vi "HFRR ADV v036.vi"() -> ()   [LabVIEW 2025] (continued)
          tunnel: [T19."Disabled" ("Disabled") T19."Enabled" ("Disabled")] -> w1363
          frame False {
          }
          frame True {
          }
        }
        n1482 = property on="About" class="Bool (strict)"("DisabledEnum"=w1363) -> ()  [unwired: 2 in, 2 out]
      }
      frame "Test Setup" {
        w1369 = T19."Enabled" ("Disabled")
        n1483 = local read "Service Password enable"() -> (w1368:bool)
        n1484 = property on="Dashboard" class="Bool (strict)"("DisabledEnum"=T19."Disabled" ("Disabled")) -> ()  [unwired: 2 in, 2 out]
        n1485 = property on="Imaging" class="Bool (strict)"("DisabledEnum"=w1369) -> ()  [unwired: 2 in, 2 out]
        n1486 = property on="Analysis" class="Bool (strict)"("DisabledEnum"=w1369) -> ()  [unwired: 2 in, 2 out]
        n1487 = property on="Home" class="Bool (strict)"("DisabledEnum"=w1369) -> ()  [unwired: 2 in, 2 out]
        n1488 = property on="Report" class="Bool (strict)"("DisabledEnum"=w1369) -> ()  [unwired: 2 in, 2 out]
        n1489 = property on="Test Setup" class="Bool (strict)"("DisabledEnum"=w1369) -> ()  [unwired: 2 in, 2 out]
        n1490 = case shown="True" w1368 {
          tunnel: [T19."Disabled" ("Disabled") T19."Enabled" ("Disabled")] -> w1367
          frame False {
          }
          frame True {
          }
        }
        n1491 = property on="About" class="Bool (strict)"("DisabledEnum"=w1367) -> ()  [unwired: 2 in, 2 out]
      }
      frame "Adv Scar" {
        w1376 = T19."Enabled" ("Disabled")
        n1492 = property on="Dashboard" class="Bool (strict)"("DisabledEnum"=T19."Disabled" ("Disabled")) -> ()  [unwired: 2 in, 2 out]
        n1493 = property on="Imaging" class="Bool (strict)"("DisabledEnum"=w1376) -> ()  [unwired: 2 in, 2 out]
        n1494 = property on="Analysis" class="Bool (strict)"("DisabledEnum"=w1376) -> ()  [unwired: 2 in, 2 out]
        n1495 = property on="Home" class="Bool (strict)"("DisabledEnum"=w1376) -> ()  [unwired: 2 in, 2 out]
        n1496 = property on="Report" class="Bool (strict)"("DisabledEnum"=w1376) -> ()  [unwired: 2 in, 2 out]
        n1497 = property on="Test Setup" class="Bool (strict)"("DisabledEnum"=w1376) -> ()  [unwired: 2 in, 2 out]
        n1498 = local read "Service Password enable"() -> (w1374:bool)
        n1499 = case shown="True" w1374 {
          tunnel: [T19."Disabled" ("Disabled") T19."Enabled" ("Disabled")] -> w1373
          frame False {
          }
          frame True {
          }
        }
        n1500 = property on="About" class="Bool (strict)"("DisabledEnum"=w1373) -> ()  [unwired: 2 in, 2 out]
      }
      frame "Calibration" {
        w1379 = T19."Enabled" ("Disabled")
        n1501 = property on="Dashboard" class="Bool (strict)"("DisabledEnum"=T19."Disabled" ("Disabled")) -> ()  [unwired: 2 in, 2 out]
        n1502 = property on="Imaging" class="Bool (strict)"("DisabledEnum"=w1379) -> ()  [unwired: 2 in, 2 out]
        n1503 = property on="Analysis" class="Bool (strict)"("DisabledEnum"=w1379) -> ()  [unwired: 2 in, 2 out]
        n1504 = property on="Home" class="Bool (strict)"("DisabledEnum"=w1379) -> ()  [unwired: 2 in, 2 out]
        n1505 = property on="Report" class="Bool (strict)"("DisabledEnum"=w1379) -> ()  [unwired: 2 in, 2 out]
        n1506 = property on="Test Setup" class="Bool (strict)"("DisabledEnum"=w1379) -> ()  [unwired: 2 in, 2 out]
        n1507 = local read "Service Password enable"() -> (w1381:bool)
        n1508 = property on="Calibration" class="Bool (strict)"("DisabledEnum"=w1379) -> ()  [unwired: 2 in, 2 out]
        n1509 = case shown="True" w1381 {
          tunnel: [T19."Disabled" ("Disabled") T19."Enabled" ("Disabled")] -> w1380
          frame False {
          }
          frame True {
          }
        }
        n1510 = property on="About" class="Bool (strict)"("DisabledEnum"=w1380) -> ()  [unwired: 2 in, 2 out]
      }
      frame "Adv Scar Report" {
        w1387 = T19."Enabled" ("Disabled")
        n1511 = property on="Dashboard" class="Bool (strict)"("DisabledEnum"=T19."Disabled" ("Disabled")) -> ()  [unwired: 2 in, 2 out]
        n1512 = property on="Imaging" class="Bool (strict)"("DisabledEnum"=w1387) -> ()  [unwired: 2 in, 2 out]
        n1513 = property on="Analysis" class="Bool (strict)"("DisabledEnum"=w1387) -> ()  [unwired: 2 in, 2 out]
        n1514 = property on="Home" class="Bool (strict)"("DisabledEnum"=w1387) -> ()  [unwired: 2 in, 2 out]
        n1515 = property on="Report" class="Bool (strict)"("DisabledEnum"=w1387) -> ()  [unwired: 2 in, 2 out]
        n1516 = property on="Test Setup" class="Bool (strict)"("DisabledEnum"=w1387) -> ()  [unwired: 2 in, 2 out]
        n1517 = local read "Service Password enable"() -> (w1386:bool)
        n1518 = case shown="True" w1386 {
          tunnel: [T19."Disabled" ("Disabled") T19."Enabled" ("Disabled")] -> w1385
          frame False {
          }
          frame True {
          }
        }
        n1519 = property on="About" class="Bool (strict)"("DisabledEnum"=w1385) -> ()  [unwired: 2 in, 2 out]
      }
      frame "Compare Files" {
        w1393 = T19."Enabled" ("Disabled")
        n1520 = local read "Service Password enable"() -> (w1392:bool)
        n1521 = property on="Dashboard" class="Bool (strict)"("DisabledEnum"=T19."Disabled" ("Disabled")) -> ()  [unwired: 2 in, 2 out]
        n1522 = property on="Imaging" class="Bool (strict)"("DisabledEnum"=w1393) -> ()  [unwired: 2 in, 2 out]
        n1523 = property on="Analysis" class="Bool (strict)"("DisabledEnum"=w1393) -> ()  [unwired: 2 in, 2 out]
        n1524 = property on="Home" class="Bool (strict)"("DisabledEnum"=w1393) -> ()  [unwired: 2 in, 2 out]
        n1525 = property on="Report" class="Bool (strict)"("DisabledEnum"=w1393) -> ()  [unwired: 2 in, 2 out]
        n1526 = property on="Test Setup" class="Bool (strict)"("DisabledEnum"=w1393) -> ()  [unwired: 2 in, 2 out]
        n1527 = case shown="True" w1392 {
          tunnel: [T19."Disabled" ("Disabled") T19."Enabled" ("Disabled")] -> w1391
          frame False {
          }
          frame True {
          }
        }
        n1528 = property on="About" class="Bool (strict)"("DisabledEnum"=w1391) -> ()  [unwired: 2 in, 2 out]
      }
      frame "Acquire" {
        n1529 = local read "Service Password enable"() -> (w1398:bool)
        n1530 = property on="Test Setup" class="Bool (strict)"("DisabledEnum"=T19."Disabled" ("Disabled")) -> ()  [unwired: 2 in, 2 out]
        n1531 = local read "Auto Start Test"() -> (w1400:bool)
        n1532 = local read "RUN"() -> (w1402:bool)
        n1533 = case shown="True" w1398 {
          tunnel: [T19."Disabled" ("Disabled") T19."Enabled" ("Disabled")] -> w1399
          frame False {
          }
          frame True {
          }
        }
        n1534 = Or(x=w1402, y=w1400) -> (x .or. y?=w1401:bool)
        n1535 = case shown="True" w1401 {
          tunnel: [T19."Enabled" ("Disabled") T19."Disabled" ("Disabled")] -> w1397
          frame False {
          }
          frame True {
          }
        }
        n1536 = property on="About" class="Bool (strict)"("DisabledEnum"=w1399) -> ()  [unwired: 2 in, 2 out]
        n1537 = property on="Imaging" class="Bool (strict)"("DisabledEnum"=w1397) -> ()  [unwired: 2 in, 2 out]
        n1538 = property on="Dashboard" class="Bool (strict)"("DisabledEnum"=w1397) -> ()  [unwired: 2 in, 2 out]
        n1539 = property on="Analysis" class="Bool (strict)"("DisabledEnum"=w1397) -> ()  [unwired: 2 in, 2 out]
        n1540 = property on="Home" class="Bool (strict)"("DisabledEnum"=w1397) -> ()  [unwired: 2 in, 2 out]
        n1541 = property on="Report" class="Bool (strict)"("DisabledEnum"=w1397) -> ()  [unwired: 2 in, 2 out]
        n1542 = property on="Calibration" class="Bool (strict)"("DisabledEnum"=w1397) -> ()  [unwired: 2 in, 2 out]
      }
      frame "About" {
        n1543 = local read "FILE"() -> (w1416:string)
        n1544 = local read "TEST FILE NAM,E SAVED"() -> (w1409:bool)
        n1545 = call <vilib>:"Trim Whitespace.vi"("string"=w1416) -> ("trimmed string"=w1415:string)  [unwired: 1 in]
        n1546 = local read "Auto Start Test"() -> (w1419:bool)
        n1547 = String Length(string=w1415) -> (length=w1414:i32)
        n1548 = Greater?(x=w1414, y=1) -> (0:w1411:bool)
        n1549 = And(x=w1411, y=w1409) -> (x .and. y?=w1410:bool)
        n1550 = local read "RUN"() -> (w1421:bool)
        n1551 = case shown="True" w1410 {
          tunnel: [T19."Disabled" ("Disabled") T19."Enabled" ("Disabled")] -> w1412
          frame False {
          }
          frame True {
          }
        }
        n1552 = Or(x=w1421, y=w1419) -> (x .or. y?=w1420:bool)
        n1553 = property on="About" class="Bool (strict)"("DisabledEnum"=T19."Enabled" ("Disabled")) -> ()  [unwired: 2 in, 2 out]
        n1554 = case shown="False" w1420 {
          tunnel: [T19."Enabled" ("Disabled") T19."Disabled" ("Disabled")] -> w1418
          frame False {
          }
          frame True {
          }
        }
        n1555 = property on="Dashboard" class="Bool (strict)"("DisabledEnum"=w1412) -> ()  [unwired: 2 in, 2 out]
        n1556 = property on="Test Setup" class="Bool (strict)"("DisabledEnum"=T19."Disabled" ("Disabled")) -> ()  [unwired: 2 in, 2 out]
        n1557 = property on="Imaging" class="Bool (strict)"("DisabledEnum"=w1418) -> ()  [unwired: 2 in, 2 out]
        n1558 = property on="Analysis" class="Bool (strict)"("DisabledEnum"=w1418) -> ()  [unwired: 2 in, 2 out]
        n1559 = property on="Home" class="Bool (strict)"("DisabledEnum"=w1418) -> ()  [unwired: 2 in, 2 out]
        n1560 = property on="Report" class="Bool (strict)"("DisabledEnum"=w1418) -> ()  [unwired: 2 in, 2 out]
      }
    }
    n1561 = local read "Quit"() -> (w1346:bool)
    "Single" <- "Single - Graph"
  }
  n1562 = disable-structure shown="Disabled" {
    disable-tunnel: [w1698 _] -> w42
    disable-tunnel: _ -> [w1697 _]
    frame Disabled {
      n1563 = while {
        tunnel: w1697 -> [_]
        tunnel: [w1699] -> w1698
        tunnel: [w1700] -> _
        i -> [w1700]
        stop <- w1699 stop-if-true
        w1716 = u16 10 items=["1.0"=10, "1.5"=15, "2.0"=20] ("stop bits (10: 1 bit)")
        n1564 = Wait (ms)(milliseconds to wait=u32 10) -> ()  [unwired: 1 out]
        n1565 = call-poly "VISA Configure Serial Port"("VISA resource name"=refnum<visa-resource-name> "ASRL1::INSTR" ("COM PORT"), "timeout (10sec)"=u32 10, "baud rate (9600)"=u32 57600, "data bits (8)"=u16 8, "stop bits (10: 1 bit)"=w1716) -> ("VISA resource name out"=w1702:refnum<visa-resource-name>, "error out"=w1711:errorcluster)  [unwired: 9 in]
        n1566 = VISA Read(VISA resource name=w1702, byte count=u32 2 ("byte count (0)")) -> (read buffer=w1710:string)  [unwired: 1 in, 3 out]
        n1567 = String Subset(string=w1710, offset (0)=0, length (rest)=2 ("length (rest)")) -> (substring=w1709:string)
        n1568 = Match Pattern(string=w1709, regular expression="<>") -> (offset past match=w1706:i32)  [unwired: 1 in, 3 out]
        n1569 = Greater Or Equal?(x=w1706, y=0) -> (x >= y?=w1701:bool)
        n1570 = case shown="True" w1701 {
          tunnel: w1702 -> [_ w1720]
          tunnel: w1711 -> [_ w1719]
          frame False {
          }
          frame True {
            n1571 = VISA Read(VISA resource name=w1720, byte count=u32 32 ("byte count (0)"), error in (no error)=w1719) -> (read buffer=w1718:string)  [unwired: 3 out]
            n1572 = String Subset(string=w1718, offset (0)=0, length (rest)=8 ("length (rest)")) -> (substring=w1722:string)
            n1573 = String Subset(string=w1718, offset (0)=8, length (rest)=8 ("length (rest)")) -> (substring=w1723:string)
            n1574 = Decimal String To Number(string=w1723) -> (number=w1730:i32)  [unwired: 2 in, 1 out]
            n1575 = Decimal String To Number(string=w1722) -> (number=w1726:i32)  [unwired: 2 in, 1 out]
            n1576 = Divide(x=w1730, y=10000) -> ()  [unwired: 1 out]
            n1577 = Divide(x=w1726, y=1000000) -> ()  [unwired: 1 out]
          }
        }
        n1578 = local read "Quit"() -> (w1699:bool)
      }
    }
    frame Enabled {
    }
  }
  n1579 = Tick Count (ms)() -> (millisecond timer value=w4:u32)
  n1580 = while {
    shift-right: [w1776] -> _
    shift-left: w6 -> [w1780]
    shift-right: [w1775] -> _
    shift-left: w5 -> [w1779]
    shift-right: [w1774] -> _
    shift-left: w6 -> [w1778]
    shift-right: [w1773] -> _
    shift-left: w5 -> [w1777]
    shift-right: [w1771] -> _
    shift-left: w4 -> [w1772]
    shift-right: [w1768] -> _
    shift-left: w3 -> [w1769]
    shift-right: [w1767] -> _
    shift-left: w3 -> [w1770]
    shift-right: [w1760] -> _
    shift-left: w3 -> [w1766]
    shift-right: [w1759] -> _
    shift-left: w3 -> [w1765]
    shift-right: [w1758] -> _
    shift-left: w3 -> [w1764]
    shift-right: [w1757] -> _
    shift-left: w3 -> [w1763]
    shift-right: [w1756] -> _
    shift-left: w3 -> [w1762]
    shift-right: [w1755] -> _
    shift-left: w3 -> [w1761]
    shift-right: [w1754] -> _
    shift-left: w3 -> [w1748]
    shift-right: [w1753] -> _
    shift-left: w3 -> [w1747]
    shift-right: [w1752] -> _
    shift-left: w3 -> [w1746]
    shift-right: [w1751] -> _
    shift-left: w3 -> [w1745]
    shift-right: [w1750] -> _
    shift-left: w3 -> [w1744]
    shift-right: [w1749] -> _
    shift-left: w3 -> [w1743]
    shift-right: [w1734] -> _
    shift-left: w3 -> [w1737]
    shift-right: [w1733] -> _
    shift-left: w3 -> [w1736]
    shift-right: [w1732] -> _
    shift-left: w3 -> [w1735]
    stop <- w1782 stop-if-true
    n1581 = local read "Read UNO"() -> (w1741:string)
    n1582 = local read "Error  2"() -> (w1781:errorcluster)
    n1583 = String Length(string=w1741) -> (length=w1740:i32)
    n1584 = call <vilib>:"Trim Whitespace.vi"("string"=w1741) -> ("trimmed string"=w1742:string)  [unwired: 1 in]
    n1585 = Greater Or Equal?(x=w1740, y=23) -> (x >= y?=w1738:bool)
    n1586 = case shown="No Error" w1781 {
      tunnel: w1780 -> [w1828 w1924]
      tunnel: w1779 -> [w1827 w1923]
      tunnel: w1778 -> [w1826 w1922]
      tunnel: w1777 -> [w1825 w1921]
      tunnel: [w1824 w1924] -> w1776
      tunnel: [w1823 w1923] -> w1775
      tunnel: [w1822 w1922] -> w1774
      tunnel: [w1821 w1921] -> w1773
      tunnel: w1772 -> [w1820 w1920]
      tunnel: [w1819 w1920] -> w1771
      tunnel: w1769 -> [w1818 w1919]
      tunnel: w1770 -> [w1817 w1918]
      tunnel: [w1816 w1919] -> w1768
      tunnel: [w1815 w1918] -> w1767
      tunnel: w1766 -> [w1814 w1917]
      tunnel: w1765 -> [w1813 w1916]
      tunnel: w1764 -> [w1812 w1915]
      tunnel: w1763 -> [w1811 w1914]
      tunnel: w1762 -> [w1810 w1913]
      tunnel: w1761 -> [w1809 w1912]
      tunnel: [w1808 w1917] -> w1760
      tunnel: [w1807 w1916] -> w1759
      tunnel: [w1806 w1915] -> w1758
      tunnel: [w1805 w1914] -> w1757
      tunnel: [w1804 w1913] -> w1756
      tunnel: [w1803 w1912] -> w1755
      tunnel: w1748 -> [w1802 w1911]
      tunnel: [w1801 w1911] -> w1754
      tunnel: [w1800 w1907] -> w1753
      tunnel: [w1799 w1906] -> w1752
      tunnel: [w1798 w1910] -> w1751
      tunnel: [w1797 w1909] -> w1750
      tunnel: [w1796 w1908] -> w1749
      tunnel: w1747 -> [w1795 w1910]
      tunnel: w1746 -> [w1794 w1909]
      tunnel: w1745 -> [w1793 w1908]
      tunnel: w1744 -> [w1792 w1907]
      tunnel: w1743 -> [w1791 w1906]
      tunnel: w1742 -> [w1790 _]
      tunnel: w1738 -> [w1789 _]
      tunnel: w1737 -> [w1788 w1905]
      tunnel: w1736 -> [w1787 w1904]
      tunnel: w1735 -> [w1786 w1903]
      tunnel: [w1785 w1905] -> w1734
      tunnel: [w1784 w1904] -> w1733
      tunnel: [w1783 w1903] -> w1732
      frame No Error {
        n1587 = case shown="True" w1789 {
          tunnel: w1828 -> [w1844 w1896]
          tunnel: w1827 -> [w1843 w1895]
          tunnel: w1826 -> [w1842 w1894]
          tunnel: w1825 -> [w1841 w1893]
          tunnel: [w1844 w1892] -> w1824
          tunnel: [w1843 w1891] -> w1823
          tunnel: [w1842 w1890] -> w1822
          tunnel: [w1841 w1889] -> w1821
          tunnel: w1820 -> [w1840 w1887]
          tunnel: [w1840 w1886] -> w1819
          tunnel: w1818 -> [w1839 w1885]
          tunnel: w1817 -> [w1838 w1884]
          tunnel: [w1839 w1883] -> w1816
          tunnel: [w1838 w1882] -> w1815
          tunnel: w1814 -> [w1837 w1881]
          tunnel: w1813 -> [w1836 w1880]
          tunnel: w1812 -> [w1835 w1879]
          tunnel: w1811 -> [w1834 w1878]
          tunnel: w1810 -> [w1833 w1877]
          tunnel: w1809 -> [w1832 w1876]
          tunnel: [w1837 w1875] -> w1808
          tunnel: [w1836 w1874] -> w1807
          tunnel: [w1835 w1873] -> w1806
          tunnel: [w1834 w1872] -> w1805
          tunnel: [w1833 w1871] -> w1804
          tunnel: [w1832 w1870] -> w1803
          tunnel: w1802 -> [w1850 w1869]
          tunnel: [w1850 w1868] -> w1801
          tunnel: [w1847 w1867] -> w1800
          tunnel: [w1846 w1866] -> w1799
          tunnel: [w1849 w1865] -> w1798
          tunnel: [w1845 w1864] -> w1797
          tunnel: [w1848 w1863] -> w1796
          tunnel: w1795 -> [w1849 w1862]
          tunnel: w1794 -> [w1848 w1861]
          tunnel: w1793 -> [w1847 w1860]
          tunnel: w1792 -> [w1846 w1859]
          tunnel: w1791 -> [w1845 w1858]
          tunnel: w1790 -> [_ w1857]
          tunnel: w1788 -> [w1831 w1856]
          tunnel: w1787 -> [w1830 w1855]
          tunnel: w1786 -> [w1829 w1854]
          tunnel: [w1831 w1853] -> w1785
          tunnel: [w1830 w1852] -> w1784
          tunnel: [w1829 w1851] -> w1783
          frame False {
          }
          frame True {
            n1588 = Tick Count (ms)() -> (millisecond timer value=w1888:u32)
            n1589 = String To Byte Array(string=w1857) -> (unsigned byte array=w1901:u8[])
            n1590 = Array Size(array=w1901) -> (size(s)=w1900:i32)
            n1591 = formula code="// --- INTERNAL VARIABLE DECLARATIONS ---\nint i = 0;\nint k = 0;\nint start_idx = -1;\nint end_idx = -1;\nint phase = 0;\nint sign0 = 1;\nint sign1 = 1;\nint ch0_val = 0;   \nint ch1_val = 0;   \nfloat ch0_raw = 0.0;\nfloat ch1_raw = 0.0;\nfloat temp0 = 0.0;\nfloat temp1 = 0.0;\nfloat ch0_clean = 0.0;\nfloat ch1_clean = 0.0;\n\nint valid_samples = 0; // FIX: Track if we actually parsed new data this window\nfloat max_allowed_bits = 8388607.0; // FIX: Change this to match your ADC max value\n\n// Temporal intermediate variables for calculation smoothing\nfloat raw_p2p_v = 0.0;\nfloat raw_friction = 0.0;\nfloat raw_cof = 0.0;\n\n// Temporal intermediate variables for Piezo voltage translations\nfloat piezo_min_v = 0.0;\nfloat piezo_max_v = 0.0;\n\n// Initialize output variables to current shift register states right away\nout_LVDT_Min_V = in_LVDT_Min_V;\nout_LVDT_Max_V = in_LVDT_Max_V;\nout_LVDT_P2P_V = in_LVDT_P2P_V;\nout_Piezo_P2P = in_Piezo_P2P;\nout_Friction_N = in_Friction_N;\nout_COF = in_COF;\nwindow_ready = 0;\n\n// --- STEP 1: PARSE EVERY STRING IN THE BYTE ARRAY ---\nif (array_size > 2) {\n    for (i = 0; i < array_size - 1; i++) {\n        if (raw_bytes[i] == 42) { // '*' character detected\n            start_idx = i;\n        }\n        \n        // Match standard delimiter sequence \";&\" or end window character\n        if (raw_bytes[i] == 59 && raw_bytes[i+1] == 38 && start_idx != -1) { \n            end_idx = i;\n            ch0_val = 0;\n            ch1_val = 0;\n            sign0 = 1;\n            sign1 = 1;\n            phase = 0; \n\n            for (k = start_idx + 1; k < end_idx; k++) {\n                if (raw_bytes[k] == 45) { // '-' sign\n                    if (phase == 0) sign0 = -1;\n                    else sign1 = -1;\n                }\n                else if (raw_bytes[k] == 43) { // '+' sign\n                    if (phase == 0) sign0 = 1;\n                    else sign1 = 1;\n                }\n                else if (raw_bytes[k] == 59) { // ';' delimiter\n                    phase = 1; \n                }\n                else if (raw_bytes[k] >= 48 && raw_bytes[k] <= 57) { // Numeric ASCII digits\n                    if (phase == 0) {\n                        ch0_val = (ch0_val * 10) + (raw_bytes[k] - 48);\n                    } else {\n                        ch1_val = (ch1_val * 10) + (raw_bytes[k] - 48);\n                    }\n                }\n            }\n\n            // Implicit type conversion\n            ch0_raw = ch0_val * sign0 * 1.0;\n            ch1_raw = ch1_val * sign1 * 1.0;\n\n            // FIX: Sanity check / Hard-clamping to catch sudden massive ASCII noise spikes\n            if (ch0_raw > max_allowed_bits)  ch0_raw = max_allowed_bits;\n            if (ch0_raw < -max_allowed_bits) ch0_raw = -max_allowed_bits;\n            if (ch1_raw > max_allowed_bits)  ch1_raw = max_allowed_bits;\n            if (ch1_raw < -max_allowed_bits) ch1_raw = -max_allowed_bits;\n\n            // --- STEP 2: 3-SAMPLE MEDIAN FILTER ---\n            m0_2 = m0_1; m0_1 = m0_0; m0_0 = ch0_raw;\n            float s0_0 = m0_0; float s0_1 = m0_1; float s0_2 = m0_2;\n            if (s0_0 > s0_1) { temp0 = s0_0; s0_0 = s0_1; s0_1 = temp0; }\n            if (s0_1 > s0_2) { temp0 = s0_1; s0_1 = s0_2; s0_2 = temp0; }\n            if (s0_0 > s0_1) { temp0 = s0_0; s0_0 = s0_1; s0_1 = temp0; }\n            ch0_clean = s0_1;\n\n            m1_2 = m1_1; m1_1 = m1_0; m1_0 = ch1_raw;\n            float s1_0 = m1_0; float s1_1 = m1_1; float s1_2 = m1_2;\n            if (s1_0 > s1_1) { temp1 = s1_0; s1_0 = s1_1; s1_1 = temp1; }\n            if (s1_1 > s1_2) { temp1 = s1_1; s1_1 = s1_2; s1_2 = temp1; }\n            if (s1_0 > s1_1) { temp1 = s1_0; s1_0 = s1_1; s1_1 = temp1; }\n            ch1_clean = s1_1;\n\n            // --- STEP 3: EXPONENTIAL FILTER (STREAM LEVEL) ---\n            if (ch0_filt == 0.0) ch0_filt = ch0_clean;\n            if (ch1_filt == 0.0) ch1_filt = ch1_clean;\n\n            ch0_filt = ch0_filt + (ch0_clean - ch0_filt) * 0.125;\n            ch1_filt = ch1_filt + (ch1_clean - ch1_filt) * 0.125;\n\n            // --- STEP 4: MIN/MAX WINDOW CONTINUOUS ACCUMULATION ---\n            if (ch0_filt > max_ch0) max_ch0 = ch0_filt;\n            if (ch0_filt < min_ch0) min_ch0 = ch0_filt;\n            if (ch1_filt > max_ch1) max_ch1 = ch1_filt;\n            if (ch1_filt < min_ch1) min_ch1 = ch1_filt;\n\n            valid_samples++; // FIX: Successfully parsed and accumulated a clean point\n            start_idx = -1; \n        }\n    }\n}\n\n// --- STEP 5: WINDOW EVALUATION ENGINE ---\n// FIX: Condition updated to verify that valid samples exist for both channels\nif (((current_time_ms - start_time_ms) >= 50) && (valid_samples > 0) && (min_ch0 < 9000000.0) && (min_ch1 < 9000000.0)) {\n    window_ready = 1;\n\n    // Linear Bit-to-Voltage Transformations (LVDT - Channel 0)\n    out_LVDT_Min_V = (min_ch0 * VREF) / 8388607.0;\n    out_LVDT_Max_V = (max_ch0 * VREF) / 8388607.0;\n    raw_p2p_v = out_LVDT_Max_V - out_LVDT_Min_V;\n\n    // Linear Bit-to-Voltage Transformations (Piezo - Channel 1)\n    piezo_min_v = (min_ch1 * VREF) / 8388607.0;\n    piezo_max_v = (max_ch1 * VREF) / 8388607.0;\n    \n    // Assign Peak-to-Peak Voltage directly to output indicator (Matches Python logic)\n    out_Piezo_P2P = piezo_max_v - piezo_min_v;\n    \n    // Force scaling calculations using Voltage delta * Newtons/Volt Factor\n    raw_friction = out_Piezo_P2P * PIEZO_CAL_FACTOR + 0.44528;\n    raw_cof = raw_friction / NORMAL_FORCE;\n\n    // --- STEP 6: OUTPUT METRIC SMOOTHING (Low-Pass Filter Alpha = 0.05) ---\n    // Seed initial historical metrics if first loop iteration\n    if (hist_LVDT_P2P == 0.0) hist_LVDT_P2P = raw_p2p_v;\n    if (hist_Friction == 0.0) hist_Friction = raw_friction;\n    if (hist_COF == 0.0)      hist_COF = raw_cof;\n\n    // Apply exponential output dampening\n    hist_LVDT_P2P = hist_LVDT_P2P + (raw_p2p_v - hist_LVDT_P2P) * 0.05;\n    hist_Friction = hist_Friction + (raw_friction - hist_Friction) * 0.05; // Note: Can drop to 0.02 for more aggressive damping\n    hist_COF      = hist_COF + (raw_cof - hist_COF) * 0.05;\n\n    // Direct smoothed parameters out to UI Indicators\n    out_LVDT_P2P_V = hist_LVDT_P2P;\n    out_Friction_N = hist_Friction;\n    out_COF        = hist_COF;\n\n    // Reset tracking targets to extreme boundaries safely\n    min_ch0 = 9999999.0;\n    max_ch0 = -9999999.0;\n    min_ch1 = 9999999.0;\n    max_ch1 = -9999999.0;\n\n    valid_samples = 0; // FIX: Reset counter for next time frame\n    start_time_ms = current_time_ms;\n}"("raw_bytes"=w1901, "array_size"=w1900, "VREF"="VREF", "PIEZO_CAL_FACTOR"="PIEZO_CAL_FACTOR", "NORMAL_FORCE"="NORMAL_FORCE", "min_ch0"=w1896, "max_ch0"=w1895, "min_ch1"=w1894, "max_ch1"=w1893, "current_time_ms"=w1888, "start_time_ms"=w1887, "ch0_filt"=w1885, "ch1_filt"=w1884, "m0_0"=w1881, "m0_1"=w1880, "m0_2"=w1879, "m1_0"=w1878, "m1_1"=w1877, "m1_2"=w1876, "in_LVDT_Min_V"=w1869, "in_LVDT_Max_V"=w1862, "in_LVDT_P2P_V"=w1861, "in_Piezo_P2P"=w1860, "in_Friction_N"=w1859, "in_COF"=w1858, "hist_LVDT_P2P"=w1856, "hist_Friction"=w1855, "hist_COF"=w1854) -> ("window_ready"=→"Valid_data":dbl, "out_LVDT_Min_V"=w1868:dbl, "out_LVDT_Max_V"=w1867:dbl, "out_LVDT_P2P_V"=w1866:dbl, "out_Piezo_P2P"=w1865:dbl, "out_Friction_N"=w1864:dbl, "out_COF"=w1863:dbl, "min_ch0"=w1892:dbl, "max_ch0"=w1891:dbl, "min_ch1"=w1890:dbl, "max_ch1"=w1889:dbl, "start_time_ms"=w1886:u32, "ch0_filt"=w1883:dbl, "ch1_filt"=w1882:dbl, "m0_0"=w1875:dbl, "m0_1"=w1874:dbl, "m0_2"=w1873:dbl, "m1_0"=w1872:dbl, "m1_1"=w1871:dbl, "m1_2"=w1870:dbl, "hist_LVDT_P2P"=w1853:dbl, "hist_Friction"=w1852:dbl, "hist_COF"=w1851:dbl)
            "LVDT MIN" <- w1868
            "LVDT MAX" <- w1867
            "LVDT Peak" <- w1866
            "pizo raw" <- w1865
            "cof" <- w1863
            "Frictioin Force Raw" <- w1864
          }
        }
      }
      frame Error {
      }
    }
    n1592 = local read "Quit"() -> (w1782:bool)
  }
  n1593 = disable-structure shown="Disabled" {
    disable-tunnel: errorcluster {"status"=TRUE, "code"=0, "source"="Init"} ("error IO") -> [w1927 _]
    disable-tunnel: [w1925 _] -> w45
    frame Disabled {
      n1594 = while {
        shift-right: [w1943] -> w1929
        shift-left: _ -> [w1934]
        shift-right: [w1942] -> w1928
        shift-left: w1927 -> [w1936]
        tunnel: [w1931] -> w1925
        tunnel: [w1941] -> _
        i -> [w1941]
        stop <- w1931 stop-if-true
        n1595 = local read "Port 1a"() -> (w1937:bool)
        n1596 = local read "Port 3"() -> (w1938:bool)
        n1597 = local read "Com Port 1"() -> (w1935:refnum<visa-resource-name>)
        n1598 = Or(x=w1938, y=w1937) -> (x .or. y?=w1940:bool)
        n1599 = Unbundle(w1936) -> ("status"=→"Port 3":bool)  [unwired: 2 out]
        n1600 = Not Equal?(x=w1935, y=w1934) -> (x != y?=w1932:bool)
        n1601 = case shown="True" w1940 {
          frame False {
            w1946 = TRUE ("Visible")
            n1602 = property on="Port 1a" class="Bool (strict)"("Visible"=w1946) -> ()  [unwired: 2 in, 2 out]
            n1603 = property on="Port 3" class="Bool (strict)"("Visible"=w1946) -> ()  [unwired: 2 in, 2 out]
          }
          frame True {
            w1947 = TRUE ("Visible")
            n1604 = property on="Port 1a" class="Bool (strict)"("Visible"=w1947) -> ()  [unwired: 2 in, 2 out]
            n1605 = property on="Port 3" class="Bool (strict)"("Visible"=w1947) -> ()  [unwired: 2 in, 2 out]
          }
        }
        n1606 = Wait (ms)(milliseconds to wait=u32 40) -> ()  [unwired: 1 out]
        n1607 = case shown="True" w1932 {
          tunnel: [w1944 errorcluster {"status"=TRUE, "code"=0, "source"="Init"} ("error out")] -> w1933
          tunnel: w1936 -> [w1944 _]
          frame False {
          }
          frame True {
          }
        }
        n1608 = case shown="Error" w1933 {
          selector: w1933 -> [w1954 w1972]
          tunnel: [w1957 w1976] -> w1943
          tunnel: [w1956 w1970] -> w1942
          tunnel: w1934 -> [w1955 w1974]
          frame No Error {
            n1609 = property class="Instr"(reference=w1955, error in=w1954) -> (reference out=w1952:refnum<visa-resource-name>, error out=w1953:errorcluster, "Serial Settings:Number of Bytes at Serial Port"=w1949:u32)
            n1610 = Greater?(x=w1949, y=u32 5) -> (0:w1948:bool)
            n1611 = Not(x=w1948) -> (.not. x?=→"Port 1a":bool)
            n1612 = while {
              tunnel: [w1965] -> w1956
              tunnel: [w1964] -> w1957
              tunnel: w1953 -> [w1963]
              tunnel: w1952 -> [w1962]
              stop <- TRUE stop-if-true
              n1613 = property class="Instr" props=["Serial Settings:Number of Bytes at Serial Port"](reference=w1962, error in=w1963) -> (reference out=w1967:refnum<visa-resource-name>, error out=w1966:errorcluster)  [unwired: 1 out]
              n1614 = VISA Read(VISA resource name=w1967, byte count=u32 50, error in (no error)=w1966) -> (VISA resource name out=w1964:refnum<visa-resource-name>, read buffer=w1959:string, error out=w1965:errorcluster)  [unwired: 1 out]
              n1615 = Wait (ms)(milliseconds to wait=u32 5) -> ()  [unwired: 1 out]
            }
          }
          frame Error {
            w1982 = u16 0 items=["None", "XON/XOFF", "RTS/CTS", "XON/XOFF & RTS/CTS", "DTR/DSR", "XON/XOFF & DTR/DSR"] ("flow control (0:none)  2")
            w1980 = u16 10 items=["1.0"=10, "1.5"=15, "2.0"=20] ("stop bits 2")
            w1978 = u16 0 items=["None", "Odd", "Even", "Mark", "Space"] ("parity 2")
            w1979 = u32 10000  # timeout (10sec)
            n1616 = VISA Close(VISA resource name=w1974, error in (no error)=w1972) -> (error out=w1975:errorcluster)
            n1617 = local write "Port 1a"(FALSE ("Port 1a")) -> ()
            n1618 = local read "Com Port 1"() -> (w1969:refnum<visa-resource-name>)
            n1619 = call <vilib>:"Clear Errors.vi"("error in (no error)"=w1975) -> ("error out"=w1973:errorcluster)  [unwired: 5 in, 1 out]
            n1620 = call-poly "VISA Configure Serial Port"("VISA resource name"=w1969, "timeout (10sec)"=w1979, "baud rate (9600)"=u32 250000 ("baud rate  2"), "data bits (8)"=u16 8 ("data bits  2"), "parity (0:none)"=w1978, "error in (no error)"=w1973, "stop bits (10: 1 bit)"=w1980, "flow control (0:none)"=w1982) -> ("VISA resource name out"=w1983:refnum<visa-resource-name>, "error out"=w1984:errorcluster)  [unwired: 6 in]
            n1621 = flat-sequence {
              tunnel: w1983 -> [w1986]
              tunnel: w1984 -> [w1985]
              tunnel: [w1986] -> w1976
              tunnel: [w1985] -> w1970
              frame #0 {
                n1622 = Wait (ms)(milliseconds to wait=u32 50) -> ()  [unwired: 1 out]
              }
            }
            "Residual Uno" <- ""
          }
        }
        n1623 = local read "Quit"() -> (w1931:bool)
        "Error Uno" <- w1936
      }
      n1624 = VISA Close(VISA resource name=w1929, error in (no error)=w1928) -> (error out=w1926:errorcluster)
      n1625 = call <vilib>:"Clear Errors.vi"("error in (no error)"=w1926) -> ()  [unwired: 5 in, 2 out]
    }
    frame Enabled {
    }
  }
  n1626 = while {
    stop <- w1997 stop-if-true
    # "V0OLTAGE TO STROKE (peice vise calibration)"
    n1627 = local read "LVDT MIN"() -> (w1989:dbl)
    n1628 = local read "LVDT Peak"() -> (w1988:dbl)
    n1629 = Wait (ms)(milliseconds to wait=u32 10) -> ()  [unwired: 1 out]
    n1630 = formula code="// Dynamic Parameterized Linear Interpolation Node\n// Inputs: vpp_val, voltages (Array), distances (Array)\n// Outputs: stroke\n\nint i = 0;\nint segments = 11; // 12 points make 11 interpolation segments\n\n// 1. Lower Boundary Clamp\nif (vpp_val <= voltages[0]) {\n    stroke = distances[0];\n}\n// 2. Upper Boundary Clamp\nelse if (vpp_val >= voltages[segments]) {\n    stroke = distances[segments];\n}\n// 3. Dynamic Segment Search Loop\nelse {\n    stroke = distances[0]; // Fallback baseline\n    for (i = 0; i < segments; i++) {\n        if (vpp_val >= voltages[i] && vpp_val <= voltages[i+1]) {\n            // Standard linear interpolation formula using array lookups\n            stroke = distances[i] + (vpp_val - voltages[i]) * (distances[i+1] - distances[i]) / (voltages[i+1] - voltages[i]);\n            break; // Segment found, safely exit the loop\n        }\n    }\n}"("vpp_val"=w1988, "voltages"="calibration values", "distances"="STROKE") -> ("stroke"=→"LVDT STROKE":dbl)
    n1631 = local read "Calibration Tare Value"() -> (w1993:dbl)
    n1632 = local read "Calibration Tare"() -> (w1991:bool)
    n1633 = Subtract(x=w1989, y=w1993) -> (x-y=→"LVDT STROKE  Calibration":dbl)
    n1634 = case shown="True" w1991 {
      selector: w1991 -> [_ w1999]
      tunnel: w1989 -> [_ w2000]
      frame False {
      }
      frame True {
        n1635 = Not(x=w1999) -> (.not. x?=w1998:bool)
        n1636 = local write "Calibration Tare"(w1998) -> ()
        "Calibration Tare Value" <- w2000
      }
    }
    n1637 = local read "Quit"() -> (w1997:bool)
  }
  n1638 = while {
    stop <- w2023 stop-if-true
    n1639 = local read "Due read"() -> (w2021:string)
    n1640 = call <vilib>:"High Resolution Polling Wait.vi"("seconds to wait"=0.02) -> ()  [unwired: 10 in, 1 out]
    n1641 = local read "Frictioin Force Raw"() -> (w2003:dbl)
    n1642 = Spreadsheet String To Array(delimiter (Tab)=";", format string="", spreadsheet string=w2021, array type (2D Dbl)=string[] []) -> (array=w2018:string[])
    n1643 = Fract/Exp String To Number(string=w2018) -> (number=w2017:dbl[])  [unwired: 3 in, 1 out]
    n1644 = call <vilib>:"Median Filter PtByPt.vi"("rank"=2, "x"=w2003) -> ("Filtered x"=→"Friction":dbl)  [unwired: 2 in, 1 out]
    n1645 = Index Array(array=w2017) -> (element #1=→"Sample Temperature":dbl, element #2=→"Target Sample Temperature":dbl, element #3=→"Current Duty Cycle":dbl, element #4=→"Ambient Temperature":dbl, element #5=→"Dac Status":dbl, element #6=→"Vpp":dbl, element #7=→"Active Error Code":dbl, element #8=→"Kp":dbl, element #9=→"Ki":dbl, element #10=→"Kd":dbl, element #11=→"SampleRaw":dbl, element #12=→"AmbRaw":dbl)  [unwired: 12 in]
    n1646 = local read "Quit"() -> (w2023:bool)
  }
  n1647 = while {
    shift-right: [w2037] -> w41
    shift-left: _ -> [w2029]
    shift-right: [w2024] -> w40
    shift-left: errorcluster {"status"=FALSE, "code"=0, "source"="Init"} ("error out") -> [w2031]
    tunnel: [w2026] -> w44
    tunnel: [w2036] -> _
    i -> [w2036]
    stop <- w2026 stop-if-true
    n1648 = local read "Com Port 2"() -> (w2030:refnum<visa-resource-name>)
    n1649 = local read "Port 2a"() -> (w2032:bool)
    n1650 = Unbundle(w2031) -> ("status"=→"Port 4":bool)  [unwired: 2 out]
    n1651 = call <vilib>:"High Resolution Polling Wait.vi"("seconds to wait"=0.02) -> ()  [unwired: 10 in, 1 out]
    n1652 = local read "Port 4"() -> (w2033:bool)
    n1653 = Not Equal?(x=w2030, y=w2029) -> (x != y?=w2028:bool)
    n1654 = Or(x=w2033, y=w2032) -> (x .or. y?=w2035:bool)
    n1655 = case shown="False" w2035 {
      frame False {
        w2040 = TRUE ("Visible")
        n1656 = property on="Port 2a" class="Bool (strict)"("Visible"=w2040) -> ()  [unwired: 2 in, 2 out]
        n1657 = property on="Port 4" class="Bool (strict)"("Visible"=w2040) -> ()  [unwired: 2 in, 2 out]
      }
      frame True {
        w2041 = TRUE ("Visible")
        n1658 = property on="Port 2a" class="Bool (strict)"("Visible"=w2041) -> ()  [unwired: 2 in, 2 out]
        n1659 = property on="Port 4" class="Bool (strict)"("Visible"=w2041) -> ()  [unwired: 2 in, 2 out]
      }
    }
    n1660 = case shown="True" w2028 {
      tunnel: [w2038 errorcluster {"status"=TRUE, "code"=0, "source"="Init"} ("error out")] -> w2027
      tunnel: w2031 -> [w2038 _]
      frame False {
      }
      frame True {
      }
    }
    n1661 = case shown="No Error" w2027 {
      selector: w2027 -> [w2054 w2085]
      tunnel: [w2047 w2090] -> w2037
      tunnel: [w2055 w2083] -> w2024
      tunnel: w2029 -> [w2056 w2088]
      frame No Error {
        n1662 = property class="Instr" props=["Serial Settings:Number of Bytes at Serial Port"](reference=w2056, error in=w2054) -> (reference out=w2048:refnum<visa-resource-name>, error out=w2053:errorcluster)  [unwired: 1 out]
        n1663 = while {
          tunnel: [w2064] -> w2049
          tunnel: [w2063] -> w2050
          tunnel: w2053 -> [w2062]
          tunnel: w2048 -> [w2061]
          tunnel: [w2060] -> _
          i -> [w2060]
          stop <- TRUE stop-if-true
          n1664 = property class="Instr" props=["Serial Settings:Number of Bytes at Serial Port"](reference=w2061, error in=w2062) -> (reference out=w2066:refnum<visa-resource-name>, error out=w2065:errorcluster)  [unwired: 1 out]
          n1665 = VISA Read(VISA resource name=w2066, byte count=u32 1000, error in (no error)=w2065) -> (VISA resource name out=w2063:refnum<visa-resource-name>, read buffer=→"Due read":string, error out=w2064:errorcluster)  [unwired: 1 out]
        }
        n1666 = local read "Due Write"() -> (w2046:string)
        n1667 = call <vilib>:"Trim Whitespace.vi"("string"=w2046) -> ("trimmed string"=w2045:string)  [unwired: 1 in]
        n1668 = Not Equal?(x=w2045, y="") -> (x != y?=w2051:bool)
        n1669 = VISA Flush I/O Buffer(VISA resource name=w2050) -> (VISA resource name out=w2043:refnum<visa-resource-name>, error out=→"error out 10":errorcluster)  [unwired: 2 in]
        n1670 = case shown="True" w2051 {
          tunnel: w2043 -> [w2068 w2073]
          tunnel: [w2068 w2077] -> w2047
          tunnel: w2049 -> [w2067 w2072]
          tunnel: [w2067 w2075] -> w2055
          tunnel: w2045 -> [_ w2071]
          tunnel: [_ w2074] -> _
          frame False {
            # "DATA  WRITE LOOP"
          }
          frame True {
            n1671 = Concatenate Strings(w2071, "\r\n") -> (w2070:string)
            n1672 = VISA Write(VISA resource name=w2073, write buffer=w2070, error in (no error)=w2072) -> (VISA resource name out=w2077:refnum<visa-resource-name>, return count=w2074:u32, error out=w2076:errorcluster)
            n1673 = flat-sequence {
              tunnel: w2076 -> [w2079]
              tunnel: [w2079] -> w2075
              frame #0 {
                n1674 = local write "Due Write"("" ("Command")) -> ()
                n1675 = Wait (ms)(milliseconds to wait=u32 5) -> ()  [unwired: 1 out]
              }
            }
          }
        }
        "Port 2a" <- TRUE ("Port 2a")
      }
      frame Error {
        w2096 = u16 0 items=["None", "XON/XOFF", "RTS/CTS", "XON/XOFF & RTS/CTS", "DTR/DSR", "XON/XOFF & DTR/DSR"] ("flow control (0:none)  2")
        w2094 = u16 10 items=["1.0"=10, "1.5"=15, "2.0"=20] ("stop bits 2")
        w2092 = u16 0 items=["None", "Odd", "Even", "Mark", "Space"] ("parity 2")
        w2093 = u32 10000  # timeout (10sec)
        n1676 = VISA Clear(VISA resource name=w2088, error in (no error)=w2085) -> (VISA resource name out=w2087:refnum<visa-resource-name>, error out=w2086:errorcluster)
        n1677 = VISA Close(VISA resource name=w2087, error in (no error)=w2086) -> (error out=w2089:errorcluster)
        n1678 = call <vilib>:"Clear Errors.vi"("error in (no error)"=w2089) -> ()  [unwired: 5 in, 2 out]
        n1679 = local write "Port 2a"(FALSE ("Port 2a")) -> ()
        n1680 = local read "Com Port 2"() -> (w2082:refnum<visa-resource-name>)
        "visa due" <- w2082
        n1681 = call-poly "VISA Configure Serial Port"("VISA resource name"=w2082, "timeout (10sec)"=w2093, "baud rate (9600)"=u32 250000 ("baud rate  2"), "data bits (8)"=u16 8 ("data bits  2"), "parity (0:none)"=w2092, "stop bits (10: 1 bit)"=w2094, "flow control (0:none)"=w2096) -> ("VISA resource name out"=w2097:refnum<visa-resource-name>, "error out"=w2098:errorcluster)  [unwired: 7 in]
        n1682 = flat-sequence {
          tunnel: w2097 -> [w2100]
          tunnel: w2098 -> [w2099]
          tunnel: [w2100] -> w2090
          tunnel: [w2099] -> w2083
          frame #0 {
            n1683 = Wait (ms)(milliseconds to wait=u32 50) -> ()  [unwired: 1 out]
          }
        }
        "Residual Due" <- ""
      }
    }
    "error out 9" <- w2024
    n1684 = local read "Quit"() -> (w2026:bool)
    "Error Due" <- w2031
  }
  n1685 = local write "FRICVALZ"(0.0 ("FRICVALZ")) -> ()
  n1686 = property on="RUN" class="Bool (strict)"("Visible"=TRUE) -> ()  [unwired: 2 in, 2 out]
  n1687 = while {
    tunnel: [w2115] -> _
    tunnel: [w2102] -> w54
    i -> [w2115]
    stop <- w2102 stop-if-true
    n1688 = local read "conststatus"() -> (w2106:dbl)
    n1689 = local read "Main Tab"() -> (w2104:T2)
    n1690 = local read "EDIT"() -> (w2121:bool)
    n1691 = local read "Rate"() -> (w2120:dbl)
    n1692 = case shown="True" w2121 {
      tunnel: [FALSE TRUE] -> _
      frame False {
      }
      frame True {
      }
    }
    n1693 = Equal?(x=w2104, y=T29."About" ("Main Tab")) -> (x = y?=w2113:bool)
    n1694 = Equal?(x=w2106, y=0.0) -> (x = y?=w2107:bool)
    n1695 = Divide(x=1.0, y=w2120) -> (x/y=w2116:dbl)
    "Time 2" <- w2116
    n1696 = case shown="True" w2107 {
      frame False {
      }
      frame True {
        # "C:\\WinDucom\\calibrate WO 2391.dcf"
        n1697 = local write "Lan flag"(22) -> ()
        n1698 = local write "conststatus"(10.0 ("rpm value : 2")) -> ()
        n1699 = String To Path(string="C:\\LAB-IQ\\calibrate WO 2465.dcf") -> (path=w2127:path)
        n1700 = Open/Create/Replace File "Open File"(file path (use dialog)=w2127) -> (refnum out=w2125:refnum<file>)  [unwired: 5 in, 2 out]
        n1701 = for {
          N: 23 -> [_]
          tunnel: w2125 -> [w2136]
          i -> [w2130]
          (unwired) TRUE ("line mode (F)")
          n1702 = Read from Text File "Read File"(file (use dialog)=w2136) -> (text=w2135:string)  [unwired: 3 in, 3 out]
          n1703 = Match Pattern(string=w2135, regular expression="]") -> (after substring=w2133:string)  [unwired: 1 in, 3 out]
          n1704 = String Subset(string=w2135, offset (0)=5, length (rest)=10 ("length (rest)")) -> (substring=w2128:string)
          n1705 = Fract/Exp String To Number(string=w2128) -> (number=w2129:dbl)  [unwired: 3 in, 1 out]
          n1706 = Match Pattern(string=w2133, regular expression="-") -> (before substring=w2131:string)  [unwired: 1 in, 3 out]
          n1707 = case shown="10" w2130 {
            tunnel: w2129 -> [_ _ _ _ _ _ _ _ _ _ w2143 _ _ _ _ _ _ _ _ _ _ _ _ _]
            tunnel: w2131 -> [_ _ _ _ w2139 w2140 w2141 _ _ _ _ _ _ _ _ _ _ _ _ _ w2144 w2145 w2146 _]
            frame 0 {
            }
            frame 1 {
            }
            frame 2 {
            }
            frame 3 {
            }
            frame 4 {
              n1708 = local write "Com Port 1"(w2139) -> ()
            }
            frame 5 {
              n1709 = local write "Com Port 2"(w2140) -> ()
              n1710 = local write "visa due"(w2140) -> ()
            }
            frame 6 {
              n1711 = String To Path(string=w2141) -> (path=w2142:path)
              n1712 = local write "File Path"(w2142) -> ()
              "String" <- w2141
            }
            frame 7 {
            }
            frame 8 {
            }
            frame 9 {
            }
            frame 10 {
              n1713 = local write "Language Selection"(w2143) -> ()
            }
            frame 11 {
            }
            frame 12 {
            }
            frame 13 {
            }
            frame 14 {
            }
            frame 15 {
            }
            frame 16 {
            }
            frame 17 {
            }
            frame 18 {
            }
            frame 21 {
            }
            frame 22 {
              n1714 = local write "Com Port 3"(w2144) -> ()
            }
            frame 20 {
              n1715 = local write "Camera Port :"(w2145) -> ()
            }
            frame 19 {
              n1716 = local write "C3 :"(w2146) -> ()
            }
            frame 23, Default {
            }
          }
        }
      }
    }
    n1717 = Select(t=u32 2500 ("milliseconds to wait"), s=w2113, f=u32 500 ("milliseconds to wait")) -> (s? t:f=w2111:u32)
    n1718 = Multiply(x=w2116, y=w2111) -> (x*y=w2118:dbl)
    n1719 = call "Elapsed Time2"("Time Target (s)"=w2118, "Auto Reset"=TRUE) -> ("Time has Elapsed"=w2108:bool)  [unwired: 10 in, 7 out]
    n1720 = case shown="True" w2108 {
      frame False {
      }
      frame True {
        n1721 = stacked-sequence {
          frame #0 {
            # "DATA PROCESSING"
            # "115 mV/N"
            n1722 = local read "Sample Temperature"() -> (w2149:dbl)
            n1723 = local read "RH Numeric:"() -> (→"Humidity ( %RH )":dbl)
            n1724 = local read "FRICVALZ"() -> (w2166:dbl)
            n1725 = local read "Friction"() -> (w2152:dbl)
            n1726 = call <vilib>:"Mean PtByPt.vi"("x"=w2149, "sample length"=100) -> ("mean"=w2148:dbl)  [unwired: 2 in, 1 out]
            "TEMP 2" <- w2148
            "TEMP 3" <- w2148
            n1727 = Subtract(x=w2152, y=w2166) -> (x-y=w2161:dbl)
            "FF 2" <- w2161
            "FF 4" <- w2161
            n1728 = local read "Ambient Temperature"() -> (→"AIR TEMP":dbl)
            n1729 = local read "TEMP"() -> (w2165:dbl)
            n1730 = local write "FF 3"(w2161) -> ()
            n1731 = Compound Arithmetic op=OR("FRICVALZ 4", "FRICVALZ 3", "FRICVALZ 2") -> (w2157:bool)
            n1732 = case shown="True" w2157 {
              tunnel: w2152 -> [_ w2172]
              frame False {
              }
              frame True {
                w2171 = FALSE ("FRICVALZ")
                n1733 = local write "FRICVALZ 3"(w2171) -> ()
                n1734 = local write "FRICVALZ 2"(w2171) -> ()
                n1735 = local write "FRICVALZ 4"(w2171) -> ()
                "FRICVALZ" <- w2172
              }
            }
            n1736 = Not A Number/Path/Refnum?(number/path/refnum=w2165) -> (NaN/Path/Refnum?=w2164:bool)
            n1737 = Not A Number/Path/Refnum?(number/path/refnum=w2161) -> (NaN/Path/Refnum?=w2163:bool)
            n1738 = Divide(x=w2161, y=1.96) -> (x/y=w2158:dbl)
            n1739 = Compound Arithmetic op=OR(w2164, w2163) -> (w2162:bool)
            n1740 = Not A Number/Path/Refnum?(number/path/refnum=w2158) -> (NaN/Path/Refnum?=w2159:bool)
            n1741 = case shown="True" w2162 {
              frame False {
              }
              frame True {
                n1742 = local write "TEMP"(0.0 ("TEMP")) -> ()
                n1743 = local write "FF 2"(0.0 ("FF 2")) -> ()
                n1744 = local write "reinit"(TRUE ("reinit")) -> ()
              }
            }
            n1745 = local write "TEMP"(w2148) -> ()
            n1746 = Select(t=0.0, s=w2159, f=w2158) -> (s? t:f=w2151:dbl)
            "COF 2" <- w2151
            n1747 = local write "COF 3"(w2151) -> ()
          }
        }
      }
    }
    n1748 = Wait (ms)(milliseconds to wait=u32 50) -> ()  [unwired: 1 out]
    n1749 = local read "Quit"() -> (w2102:bool)
    "Rate" <- 2500.0 ("No of Samples")
  }
  n1750 = while {
    tunnel: [w2192] -> _
    tunnel: [w2175] -> w56
    tunnel: w1 -> [_]
    i -> [w2192]
    stop <- w2175 stop-if-true
    # "C:\\LAB-IQ-NXT\\Scar View.exe"
    n1751 = local read "OK Button 16"() -> (w2182:bool)
    n1752 = local read "Main Tab"() -> (w2176:T2)
    n1753 = local read "service 3"() -> (w2177:bool)
    n1754 = local read "OPEN 6"() -> (w2179:bool)
    n1755 = local read "EDIT 2"() -> (w2181:bool)
    n1756 = flat-sequence {
      frame #0 {
        n1757 = stacked-sequence {
          frame #0 {
            n1758 = local read "EDIT"() -> (w2670:bool)
            n1759 = case shown="False" w2670 {
              tunnel: [u8 2 ("Disabled") u8 0 ("Disabled")] -> _
              frame False {
                w2672 = FALSE
                n1760 = local write "Password"("") -> ()
                n1761 = local write "x = y?"(w2672) -> ()
                n1762 = property on="Password" class="Str"("Visible"=w2672) -> ()  [unwired: 2 in, 2 out]
              }
              frame True {
                n1763 = property on="Password" class="Str"("Visible"=TRUE) -> ()  [unwired: 2 in, 2 out]
              }
            }
            "dipl pwd" <- "@143$\n" ("dipl pwd")
          }
          frame #1 {
          }
          frame #2 {
          }
          frame #3 {
          }
          frame #4 {
            n1764 = String To Byte Array(string="Password") -> (unsigned byte array=w2683:u8[])
            n1765 = Search 1D Array(1D array=w2683, element=u8 10) -> (index of element=w2681:i32)  [unwired: 1 in]
            n1766 = Index Array(array=w2683, index=w2681) -> (element=w2682:u8)
            n1767 = Equal?(x=w2682, y=10) -> (x = y?=w2678:bool)
            n1768 = case shown="True" w2678 {
              frame False {
              }
              frame True {
                # "password"
                # "password"
                n1769 = local read "Password"() -> (w2695:string)
                n1770 = String To Byte Array(string=w2695) -> (unsigned byte array=w2698:u8[])
                n1771 = String To Byte Array(string="@143$\n") -> (unsigned byte array=w2685:u8[])
                n1772 = Array Size(array=w2698) -> (size(s)=w2694:i32)
                n1773 = Array Size(array=w2685) -> (size(s)=w2690:i32)
                n1774 = for {
                  N: w2694 -> [_]
                  tunnel: w2698 -> [w2711]
                  tunnel: [w2709] -> w2699 mode=indexing
                  tunnel: w2694 -> [w2706]
                  i -> [w2707]
                  n1775 = Decrement(x=w2706) -> (x-1=w2705:i32)
                  n1776 = Index Array(array=w2711, index=w2707) -> (element=w2710:u8)
                  n1777 = Equal?(x=w2707, y=w2705) -> (x = y?=w2704:bool)
                  n1778 = Number To Decimal String(number=w2710) -> (decimal integer string=w2708:string)  [unwired: 1 in]
                  n1779 = Select(t="", s=w2704, f="\r") -> (s? t:f=w2701:string)
                  n1780 = Concatenate Strings(w2708, w2701) -> (w2709:string)
                }
                n1781 = for {
                  N: w2690 -> [_]
                  tunnel: w2685 -> [w2722]
                  tunnel: [w2720] -> w2688 mode=indexing
                  tunnel: w2690 -> [w2717]
                  i -> [w2718]
                  n1782 = Decrement(x=w2717) -> (x-1=w2716:i32)
                  n1783 = Index Array(array=w2722, index=w2718) -> (element=w2721:u8)
                  n1784 = Equal?(x=w2718, y=w2716) -> (x = y?=w2715:bool)
                  n1785 = Number To Decimal String(number=w2721) -> (decimal integer string=w2719:string)  [unwired: 1 in]
                  n1786 = Select(t="", s=w2715, f="\r") -> (s? t:f=w2712:string)
                  n1787 = Concatenate Strings(w2719, w2712) -> (w2720:string)
                }
                n1788 = local read "file path"() -> (w2684:path)
                n1789 = call <vilib>:"Read Characters From File.vi"("file path (dialog if empty)"=w2684) -> ("character string"=w2697:string)  [unwired: 5 in, 3 out]
                "string" <- w2697
                n1790 = flat-sequence {
                  tunnel: [w2700] -> _
                  frame #0 {
                    w2700 = ""
                    n1791 = local write "Password"(w2700) -> ()
                  }
                }
                n1792 = Concatenate Strings(w2688) -> (w2689:string)
                n1793 = Concatenate Strings(w2697) -> (w2696:string)
                n1794 = Concatenate Strings(w2699) -> (w2692:string)
                n1795 = Equal?(x=w2692, y=w2696) -> (x = y?=w2687:bool)
                n1796 = Equal?(x=w2692, y=w2689) -> (x = y?=w2693:bool)
                n1797 = Or(x=w2687, y=w2693) -> (x .or. y?=→"x = y?":bool)
              }
            }
          }
        }
        n1798 = local read "x = y?"() -> (w2668:bool)
        n1799 = And(x="EDIT", y=w2668) -> (x .and. y?=w2666:bool)
        n1800 = case shown="True" w2666 {
          tunnel: [u8 2 ("Disabled") u8 0 ("Disabled")] -> w2665
          tunnel: [w2872 TRUE ("Visible")] -> w2664
          frame False {
            w2872 = FALSE ("Visible")
            n1801 = local write "EDIT 2"(w2872) -> ()
          }
          frame True {
          }
        }
        n1802 = case shown="True" "SAVE" {
          frame False {
          }
          frame True {
            n1803 = stacked-sequence {
              seq-local: [w2727 _ _] -> [_ w2868 _]
              frame #0 {
                w2723 = 0.0 ("number")
                w2724 = 0.0 ("number")
                (unwired) i16 5 ("precision (6)")
                # "[CH1]    - FF\n[CH2]   - TEMPERATURE\n[CH3]    - Humidity\n[CH4]    - AIR TEMP\n[CH5]\\- Visa Uno\n[CH6] \\- Visa Due\n[CH7]  \\- file path\n[CH8]   - Displacement Gain\n[CHA]   - Stroke Gain\n[CHB]   - Stroke PID Gain\n[CHC]   -Language Selection\n[CHD]   -Power +\n[CHE]   -Power_\n[CHF]   -Heater\n[CHG]   -Humidity Wet\n[CHH]   -Humidity Dry\n[CHI]   -Integral Time"
                n1804 = local read "Language Selection"() -> (w2770:enum16{"English", "Russian"})
                n1805 = Path To String(path="File Path") -> (string=w2786:string)
                n1806 = Number To Fractional String(number=w2723, width (-)=i16 10 ("precision (6)"), precision (6)=i16 5) -> (F-format string=w2777:string)  [unwired: 1 in]
                n1807 = Number To Fractional String(number=w2770, width (-)=i16 10 ("precision (6)"), precision (6)=i16 5) -> (F-format string=w2766:string)  [unwired: 1 in]
                n1808 = Number To Fractional String(number=w2724, width (-)=i16 10 ("precision (6)"), precision (6)=i16 5) -> (F-format string=w2760:string)  [unwired: 1 in]
                n1809 = Number To Fractional String(number=w2724, width (-)=i16 10 ("precision (6)"), precision (6)=i16 5) -> (F-format string=w2757:string)  [unwired: 1 in]
                n1810 = Number To Fractional String(number=w2724, width (-)=i16 10 ("precision (6)"), precision (6)=i16 5) -> (F-format string=w2752:string)  [unwired: 1 in]
                n1811 = Number To Fractional String(number=w2724, width (-)=i16 10 ("precision (6)"), precision (6)=i16 5) -> (F-format string=w2749:string)  [unwired: 1 in]
                n1812 = Number To Fractional String(number=w2724, width (-)=i16 10 ("precision (6)"), precision (6)=i16 5) -> (F-format string=w2744:string)  [unwired: 1 in]
                n1813 = local read "Com Port 1"() -> (w2726:refnum<visa-resource-name>)
                n1814 = local read "Com Port 2"() -> (w2725:refnum<visa-resource-name>)
                n1815 = Concatenate Strings(w2786, "\\" ("string")) -> (w2785:string)
                n1816 = Number To Fractional String(number=w2723, width (-)=i16 10 ("precision (6)"), precision (6)=i16 5) -> (F-format string=w2818:string)  [unwired: 1 in]
                n1817 = Number To Fractional String(number=w2723, width (-)=i16 10 ("precision (6)"), precision (6)=i16 5) -> (F-format string=w2817:string)  [unwired: 1 in]
                n1818 = Number To Fractional String(number=w2723, width (-)=i16 10 ("precision (6)"), precision (6)=i16 5) -> (F-format string=w2811:string)  [unwired: 1 in]
                n1819 = Number To Fractional String(number=w2723, width (-)=i16 10 ("precision (6)"), precision (6)=i16 5) -> (F-format string=w2805:string)  [unwired: 1 in]
                n1820 = Number To Fractional String(number=w2723, width (-)=i16 10 ("precision (6)"), precision (6)=i16 5) -> (F-format string=w2778:string)  [unwired: 1 in]
                n1821 = Concatenate Strings("[CHA]" ("string"), w2777, "- Stroke Gain" ("string"), "\r") -> (w2771:string)
                n1822 = Concatenate Strings("[CHC]" ("string"), w2766, "-Language Selection" ("string"), "\r") -> (w2763:string)
                n1823 = Concatenate Strings("[CHD]" ("string"), w2760, "-Power +" ("string"), "\r") -> (w2742:string)
                n1824 = Concatenate Strings("[CHG]" ("string"), w2749, "-Humidity Wet" ("string"), "\r") -> (w2739:string)
                n1825 = Concatenate Strings("[CHH]" ("string"), w2744, "-Humidity Dry" ("string"), "\r") -> (w2738:string)
                n1826 = Concatenate Strings("[CH1]" ("string"), w2818, " - FF" ("string"), "\r") -> (w2816:string)
                n1827 = Concatenate Strings("[CH2]" ("string"), w2817, " - TEMPERATURE" ("string"), "\r") -> (w2815:string)
                n1828 = Concatenate Strings("[CH3]" ("string"), w2811, " - Humidity" ("string"), "\r") -> (w2808:string)
                n1829 = Concatenate Strings("[CH4]" ("string"), w2805, " - AIR TEMP" ("string"), "\r") -> (w2801:string)
                n1830 = Concatenate Strings("[CH5]" ("string"), w2726, "- Visa Uno" ("string"), "\r") -> (w2794:string)
                n1831 = Concatenate Strings("[CH6]" ("string"), w2725, "- Visa Due" ("string"), "\r") -> (w2789:string)
                n1832 = Concatenate Strings("[CH7]" ("string"), w2785, "- file path" ("string"), "\r") -> (w2788:string)
                n1833 = Concatenate Strings("[CH8]" ("string"), w2778, "- Displacement Gain" ("string"), "\r") -> (w2781:string)
                n1834 = Concatenate Strings("[CHE]" ("string"), w2757, "-Power_" ("string"), "\r") -> (w2741:string)
                n1835 = Concatenate Strings("[CHF]" ("string"), w2752, "-Heater" ("string"), "\r") -> (w2740:string)
                n1836 = Concatenate Strings(w2816, w2815, w2808, w2801, w2794, w2789, w2788, w2781, w2771, w2763, w2742, w2741, w2740, w2739, w2738) -> (w2727:string)
                "gain" <- w2727
              }
              frame #1 {
                w2829 = 0.0 ("number")
                n1837 = local read "Camera Port :"() -> (w2832:string)
                n1838 = local read "C3 :"() -> (w2840:refnum<visa-resource-name>)
                n1839 = local read "Com Port 3"() -> (w2841:refnum<visa-resource-name>)
                n1840 = Concatenate Strings("[CH8]" ("string"), w2832, "- Visa Camera" ("string"), "\r") -> (w2831:string)
                n1841 = Concatenate Strings("[CH7]" ("string"), w2840, "- Visa Humidity" ("string"), "\r") -> (w2836:string)
                n1842 = Number To Fractional String(number=w2829, width (-)=i16 10 ("precision (6)"), precision (6)=i16 5) -> (F-format string=w2856:string)  [unwired: 1 in]
                n1843 = Concatenate Strings("[CHL]" ("string"), w2841, "- Visa humid" ("string"), "\r") -> (w2844:string)
                n1844 = Number To Fractional String(number=w2829, width (-)=i16 10 ("precision (6)"), precision (6)=i16 5) -> (F-format string=w2863:string)  [unwired: 1 in]
                n1845 = Concatenate Strings("[CHK]" ("string"), w2856, "-TEMP INTERCEPT" ("string"), "\r") -> (w2852:string)
                n1846 = Concatenate Strings("[SNO]" ("string"), "" ("string"), "-" ("string"), "\r") -> (w2849:string)
                n1847 = Concatenate Strings("[CHJ]" ("string"), w2863, "-AIR TEMP INTERCEPT" ("string"), "\r") -> (w2853:string)
                n1848 = String To Path(string="C:\\LAB-IQ\\calibrate WO 2465.dcf") -> (path=w2842:path)
                n1849 = Concatenate Strings(w2868, w2853, w2852, w2849, w2844, w2836, w2831) -> (w2867:string)
                n1850 = call <vilib>:"Write Characters To File.vi"("append to file? (new file:F)"=FALSE, "character string"=w2867, "file path (dialog if empty)"=w2842) -> ()  [unwired: 2 in, 1 out]
              }
              frame #2 {
                n1851 = local write "Lan flag"(0.0 ("Lan flag")) -> ()
                n1852 = local write "conststatus"(0.0 ("rpm value : 2")) -> ()
                n1853 = local write "SAVE"(FALSE ("OK Button 14")) -> ()
              }
            }
          }
        }
        n1854 = property on="EDIT 2" class="Bool (strict)"("Visible"=w2664) -> ()  [unwired: 2 in, 2 out]
        n1855 = property on="SAVE" class="Bool (strict)"("Visible"=w2664) -> ()  [unwired: 2 in, 2 out]
        n1856 = property on="visa due" class="CmbBox"("Disabled"=w2665) -> ()  [unwired: 2 in, 2 out]
        n1857 = property on="File Path" class="Path"("Disabled"=w2665) -> ()  [unwired: 2 in, 2 out]
        n1858 = property on="Language Selection" class="Enum (strict)"("Visible"=w2664) -> ()  [unwired: 2 in, 2 out]
        n1859 = property on="SPEED OUT:" class="DigNum (strict)"("Disabled"=w2665) -> ()  [unwired: 2 in, 2 out]
      }
    }
    n1860 = local read "RUN"() -> (w2191:bool)
    n1861 = local read "RUN"() -> (w2189:bool)
    n1862 = case shown="True" "EDIT 3" {
      frame False {
      }
      frame True {
        n1863 = local write "EDIT 3"(FALSE ("EDIT 3")) -> ()
        n1864 = local write "Main Tab"(T2."About" ("Main Tab")) -> ()
      }
    }
    n1865 = case shown="False" w2191 {
      frame False {
        n1866 = local read "stopT"() -> (w2879:bool)
        n1867 = case shown="True" w2879 {
          frame False {
          }
          frame True {
            n1868 = local write "stopT"(FALSE) -> ()
          }
        }
      }
      frame True {
        "stopT" <- TRUE
      }
    }
    n1869 = case shown="False" w2189 {
      frame False {
      }
      frame True {
      }
    }
    n1870 = case shown="True" w2181 {
      frame False {
        n1871 = property on="Password 2" class="Str"("Visible"=FALSE) -> ()  [unwired: 2 in, 2 out]
        n1872 = local write "Password 2"("" ("Password")) -> ()
      }
      frame True {
        n1873 = property on="Password 2" class="Str"("Visible"=TRUE) -> ()  [unwired: 2 in, 2 out]
        n1874 = Equal?(x="Password 2", y="HFRR1234") -> (x = y?=w2204:bool)
        n1875 = case shown="True" w2204 {
          tunnel: "Password 2" -> [w2207 _]
          frame False {
            n1876 = String Length(string=w2207) -> (length=w2208:i32)
            n1877 = Greater Than 0?(x=w2208) -> (x > 0?=w2206:bool)
            n1878 = case shown="False" w2206 {
              frame False {
                n1879 = property on="Password 2" class="Str"("Caption.Text"="Password (Advance Setting)") -> ()  [unwired: 2 in, 2 out]
              }
              frame True {
                n1880 = property on="Password 2" class="Str"("Caption.Text"="Incorrect Password!") -> ()  [unwired: 2 in, 2 out]
              }
            }
          }
          frame True {
            n1881 = local write "EDIT 2"(FALSE ("EDIT 2")) -> ()
            n1882 = local write "Password 2"("" ("Password")) -> ()
            n1883 = local write "Main Tab"(T2."Advance" ("Main Tab")) -> ()
